vi "InitApp.vi"(8 "error in":errorcluster) -> (0 "error out":errorcluster)   [LabVIEW 2012]
uses:
  <vilib>/Utility/config.llb/Read Key (String).vi
  GlobalVariables/MachineInfos.vi
  GlobalVariables/AppState.vi
  GlobalVariables/CurrentPressure.vi
  GlobalVariables/AllowContinuousPressureAcquisition.vi
  GlobalVariables/SamplesData.vi
  GlobalVariables/Samples.vi
  GlobalVariables/MeasureExportStrings.vi
  GlobalVariables/CalibrationState.vi
  GlobalVariables/SystemParameters.vi
  GlobalVariables/LanguagesSettings.vi
  <vilib>/Utility/config.llb/NI_LVConfig.lvlib
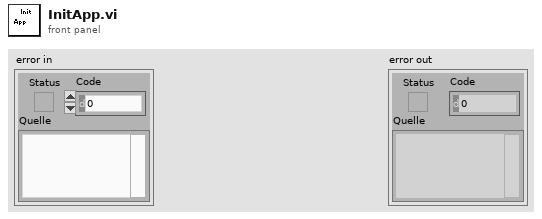
[diagram p1: front panel]
types:
  T1 = cluster{cluster{"PressureSamples":dbl[], "PressureSamples 2":dbl[]}, cluster{"PressureSamples":dbl[], "PressureSamples 2":dbl[]}}
  T2 = cluster{"date":string, "sampleNumber":string, "sampleID":string, "sampleDepth":string, "dryWeight":string, "grainDensity":string, "bulkVolume":string, "poreVolume":string, "porosity":string, "sleeveVolume":string, "sleeveLength":string, "sleeveDiameter":string, "sleeveThickness":string, "temperature":string, "comments":string}[]
  T3 = typedef "NI_LVConfig.lvlib/Config Data RefNum.ctl" = refnum<k1>
  T4 = cluster{bool, "CalibrationStep":u32, "Volumes":dbl[], "PressureRatios":dbl[]}
  T5 = cluster{"defaultLanguage":string, "languageFile":string, "languages":string, "HardwarePresent":bool}
  T6 = cluster{"Indices":u32[], "LocalizedWords":string[][]}
  T7 = cluster{"Slices":string[], "defaultLanguage":string, i32, "LocalisationFileContent[out]":cluster{"Indices":u32[], "LocalizedWords":string[][]}}
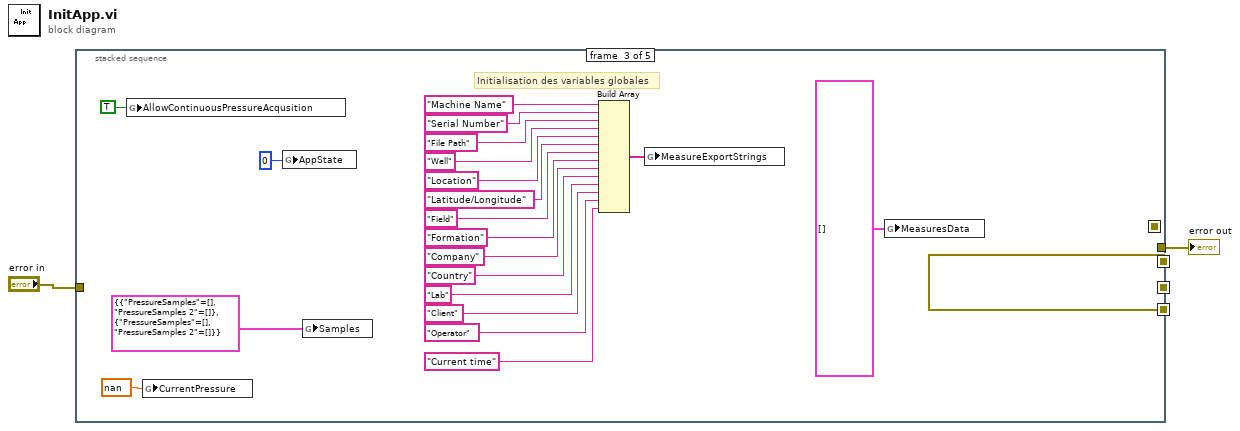
[diagram p0: block diagram]
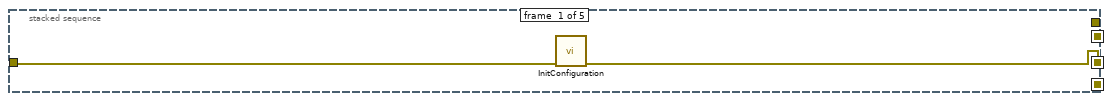
[diagram p2: hidden frame]
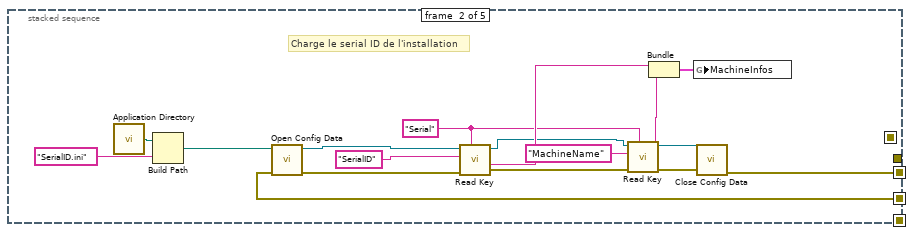
[diagram p3: hidden frame]
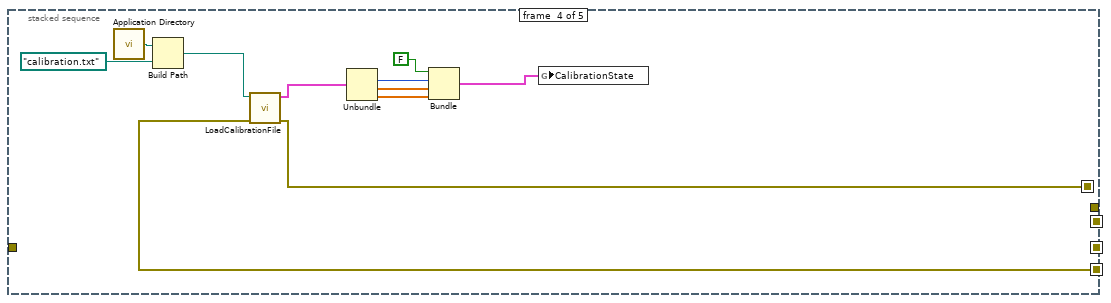
[diagram p4: hidden frame]
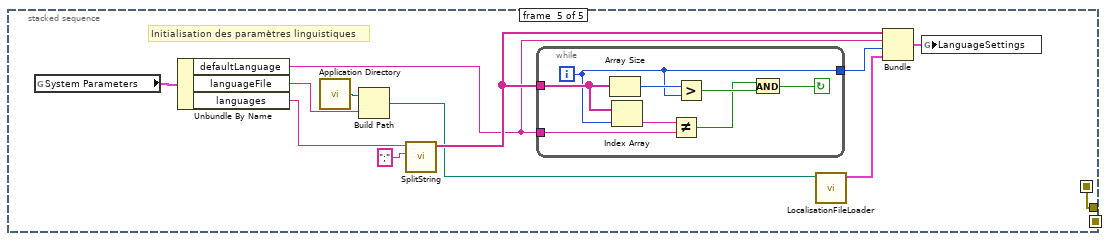
[diagram p5: hidden frame]
diagram:
  n1 = stacked-sequence {
    seq-local: [w3 _ _ _ _] -> [_ w16 _ _ _]
    seq-local: [_ w15 _ _ _] -> [_ _ w23 _ _]
    seq-local: [_ _ w23 _ _] -> [_ _ _ w49 _]
    seq-local: [_ _ _ w50 _] -> [_ _ _ _ w55]
    tunnel: "error in" -> [w4 _ _ _ _]
    tunnel: [_ _ _ _ w55] -> w1
    frame #0 {
      n2 = call "InitConfiguration.vi"("error in"=w4) -> ("error out"=w3:errorcluster)  [unwired: 10 in]
    }
    frame #1 {
      w8 = "Serial"
      # "Charge le serial ID de l'installation"
      n3 = call <vilib>:"Application Directory.vi"() -> ("Application Directory"=w19:path)
      n4 = Build Path(base path=w19, name or relative path="SerialID.ini") -> (appended path=w18:path)
      n5 = call <vilib>:"Open Config Data.vi"("error in (no error)"=w16, "configuration file path"=w18) -> ("error out"=w21:errorcluster, "refnum"=w20:T3)  [unwired: 7 in, 1 out]
      n6 = call-poly <vilib>:"Read Key.vi"("section"=w8, "error in (no error)"=w21, "key"="SerialID", "refnum"=w20) -> ("error out"=w10:errorcluster, "value"=w12:string, "refnum out"=w5:T3)  [unwired: 4 in, 1 out]
      n7 = call-poly <vilib>:"Read Key.vi"("section"=w8, "error in (no error)"=w10, "key"="MachineName", "refnum"=w5) -> ("error out"=w11:errorcluster, "value"=w9:string, "refnum out"=w6:T3)  [unwired: 4 in, 1 out]
      n8 = Bundle("value"=w12, "value"=w9) -> (w13:cluster{"value":string, "value":string})  [unwired: 1 in]
      n9 = global write "MachineInfos.vi" "MachineInfos"(w13) -> ()
      n10 = call <vilib>:"Close Config Data.vi"("error in (no error)"=w11, "refnum"=w6) -> ("error out"=w15:errorcluster)  [unwired: 8 in, 1 out]
    }
    frame #2 {
      # "Initialisation des variables globales"
      n11 = global write "AllowContinuousPressureAcquisition.vi" "AllowContinuousPressureAcqusition"(TRUE) -> ()
      n12 = global write "CurrentPressure.vi" "CurrentPressure"(nan) -> ()
      n13 = global write "AppState.vi" "AppState"(u16 0 ("MachineState")) -> ()
      n14 = global write "Samples.vi" "Samples"(T1 {{"PressureSamples"=[], "PressureSamples 2"=[]}, {"PressureSamples"=[], "PressureSamples 2"=[]}} ("PressureAndTimeSamples")) -> ()
      n15 = Build Array("Machine Name", "Serial Number" ("element"), "File Path" ("element"), "Well" ("element"), "Location", "Latitude/Longitude", "Field", "Formation", "Company", "Country", "Lab", "Client", "Operator", "Current time") -> (w22:string[])
      n16 = global write "MeasureExportStrings.vi" "MeasureExportStrings"(w22) -> ()
      n17 = global write "SamplesData.vi" "MeasuresData"(T2 [] ("MeasuresData")) -> ()
    }
    frame #3 {
      n18 = call <vilib>:"Application Directory.vi"() -> ("Application Directory"=w52:path)
      n19 = Build Path(base path=w52, name or relative path=path "calibration.txt" ("default name")) -> (appended path=w51:path)
      n20 = call "LoadCalibrationFile.vi"("error in (no error)"=w49, "Path"=w51) -> ("error out"=w50:errorcluster, "CalibrationState"=w48:T4)  [unwired: 8 in]
      n21 = Unbundle(w48) -> ("CalibrationStep"=w44:u32, "Volumes"=w45:dbl[], "PressureRatios"=w46:dbl[])  [unwired: 1 out]
      n22 = Bundle(FALSE, "CalibrationStep"=w44, "Volumes"=w45, "PressureRatios"=w46) -> (w47:T4)  [unwired: 1 in]
      n23 = global write "CalibrationState.vi" "CalibrationState"(w47) -> ()
    }
    frame #4 {
      # "Initialisation des paramètres linguistiques"
      n24 = global read "SystemParameters.vi" "System Parameters"() -> (w58:T5)
      n25 = Unbundle By Name(w58) -> ("defaultLanguage"=w56:string, "languageFile"=w57:string, "languages"=w54:string)
      n26 = call <vilib>:"Application Directory.vi"() -> ("Application Directory"=w65:path)
      n27 = Build Path(base path=w65, name or relative path=w57) -> (appended path=w60:path)
      n28 = call "SplitString.vi"("Separator"=";", "String[in]"=w54) -> ("Slices"=w62:string[])  [unwired: 9 in]
      n29 = while {
        tunnel: w62 -> [w68]
        tunnel: w56 -> [w67]
        tunnel: [w66] -> w61
        i -> [w66]
        stop <- w73 continue-if-true
        n30 = Array Size(array=w68) -> (size(s)=w71:i32)
        n31 = Index Array(array=w68, index=w66) -> (element=w69:string)
        n32 = Not Equal?(x=w69, y=w67) -> (x != y?=w70:bool)
        n33 = Greater?(x=w71, y=w66) -> (0:w72:bool)
        n34 = And(x=w70, y=w72) -> (x .and. y?=w73:bool)
      }
      n35 = call "LocalisationFileLoader.vi"("FilePath"=w60) -> ("LocalisationFileContent[out]"=w59:T6)  [unwired: 10 in]
      n36 = Bundle("Slices"=w62, "defaultLanguage"=w56, w61, "LocalisationFileContent[out]"=w59) -> (w64:T7)  [unwired: 1 in]
      n37 = global write "LanguagesSettings.vi" "LanguageSettings"(w64) -> ()
    }
  }
  "error out" <- w1
